vi "String to Type.vi"(7 "application reference (local)":refnum<vi>, 8 "Error In":errorcluster, 11 "String":string) -> (0 "Error Out":errorcluster, 2 "Rest of the String":string, 3 "Type":variant)   [LabVIEW 2015, in "Scripting.lvlib"]
uses:
  Scripting.lvlib
  <vilib>/Utility/Data Type/Type Definitions/Data Type.ctl
  <vilib>/fxp/LVFixedPointRepBitsTypeDef.ctl
  <vilib>/fxp/LVFixedPointRepRangeTypeDef.ctl
  <vilib>/Utility/Data Type/Type Definitions/Refnum Type.ctl
  <vilib>/Utility/Data Type/Type Definitions/VI Info.ctl
  <vilib>/Utility/Data Type/Type Definitions/Tag Type.ctl
  <vilib>/Utility/Data Type/NI_Data Type.lvlib
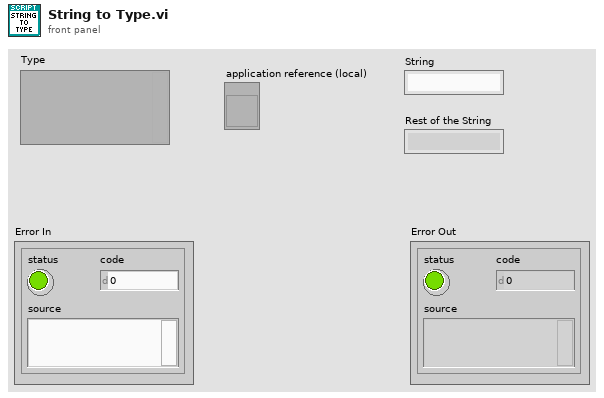
[diagram p1: front panel]
types:
  T1 = typedef "NI_Data Type.lvlib/Data Type.ctl" = enum8{"Invalid Type", "Void", "I8", "I16", "I32", "I64", "U8", "U16", "U32", "U64", "Single Float", "Double Float", "Extended Float", "Single Complex", "Double Complex", "Extended Complex", "Enum U8", "Enum U16", "Enum U32", "Enum U64", "Single Float With Unit", "Double Float With Unit", "Extended Float With Unit", "Single Complex with Unit", "Double Complex with Unit", "Extended Complex with Unit", "Boolean", "String", "Path", "Picture", "Tag", "Array", "Cluster", "Variant", "LV Variant", "Waveform", "Timestamp", "Digital Waveform", "Digital Data", "ExpressData", "Refnum", "External Data", "VI", "Poly VI", "LabVIEW Class Instance", "Fixed Point"}
  T2 = cluster{"Unit Type":enum8{"Radians", "Steradians", "Seconds", "Meters", "Kilograms", "Amperes", "Kelvins", "Moles", "Candelas", "InvalidUnit"}, "Exponent":i8}[]
  T3 = typedef "LVFixedPointRepBitsTypeDef.ctl" = cluster{"Signed":bool, "Word Length":u32, "Integer Word Length":i32}
  T4 = typedef "LVFixedPointRepRangeTypeDef.ctl" = cluster{"Range Min":dbl, "Range Max":dbl, "Delta":dbl}
  T5 = cluster{"FXP Representation":T3, "FXP Range":T4, "Include Overflow Status?":bool}
  T6 = typedef "NI_Data Type.lvlib/Refnum Type.ctl" = enum16{"NotARefnum", "UnknownRefnum", "Generic", "Datalog", "ByteStream", "Device", "Occurence", "TCPNetConnection", "Auto", "Menu", "Imaq", "Hardware", "DataSocket", "Visa", "IVI", "UDPNetConnection", "Notifier", "Queue", "Irda", "EventReg", "DotNet", "UserEvent", "Callback", "UNUSED_EMPTY_POSITION", "BlueToothNetConnection", "LVObjApp", "LVObjVI", "LVObjUnknown", "GenericClass", "UserDefinedRefnumTag", "DataValue", "RT FIFO", "TDMS File"}
  T7 = typedef "NI_Data Type.lvlib/VI Info.ctl" = cluster{"Connector Pane Pattern":i16, "Connector Pane Rotation":i16, "Flags":u32[], "Modification Date":timestamp, "Asynchronous":bool, "Non-Function":bool, "Subroutine":bool, "SubSystem":bool}
  T8 = typedef "NI_Data Type.lvlib/Tag Type.ctl" = enum16{"kNoTagType", "\tkDSCTagType", "\tkOldDAQTagType", "\tkIVITagType", "\tkVISATagType", "\tkGenClassTagType", "\tkUnusedTagType1", "\tkFPTagType", "\tkMotionTagType", "\tkDAQmxTaskTagType", "\tkDAQmxChannelTagType", "\tkDAQmxScaleTagType", "\tkDAQmxDeviceTagType", "\tkDAQmxTerminalTagType", "\tkDAQmxPhysChanTagType", "\tkDAQmxTriggerTagType", "\tkDAQmxSwitchTagType", "\tkDAQmxSignalTagType", "\tkUnusedTagType2", "\tkCANTaskTagType", "\tkCANInterfaceTagType", "\tkCANChannelTagType", "\tkNumTagTypes"}
  T9 = cluster{"Type":enum8{"Variable", "Fixed", "Bounded"}, "Size":u32}[]
  T10 = cluster{"string":string, string, "string":string}
  T11 = typedef "NI_Data Type.lvlib/Type Definition Info.ctl" = cluster{"Name":string, "Timestamp":u32}
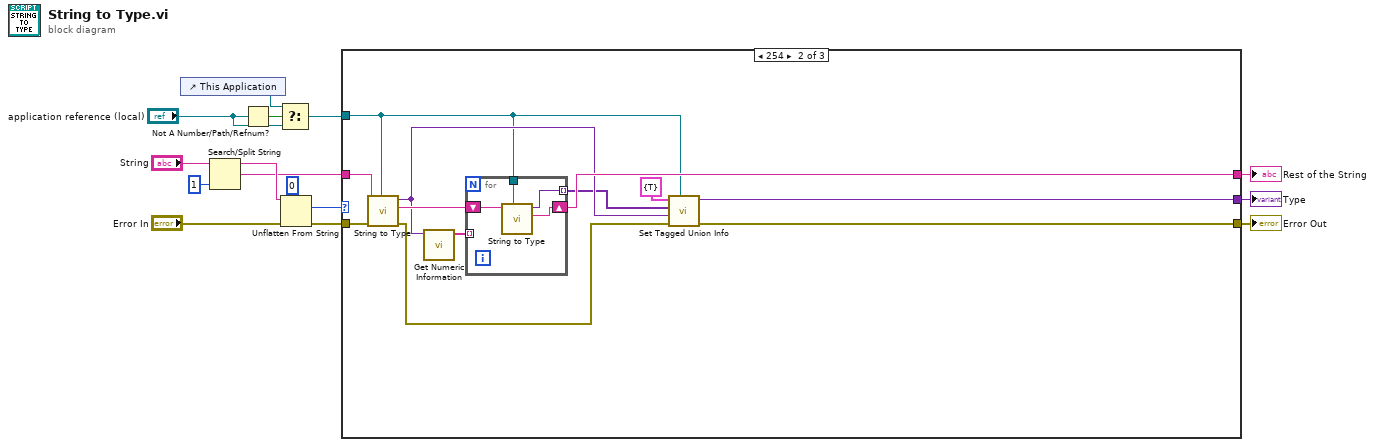
[diagram p0: block diagram]
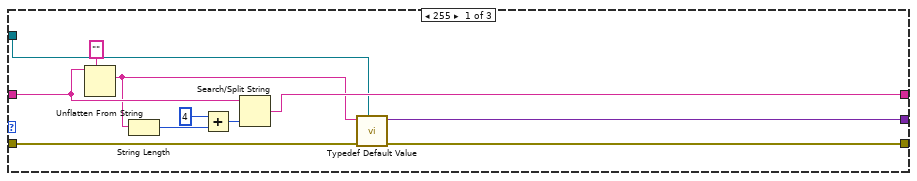
[diagram p2: hidden frame]
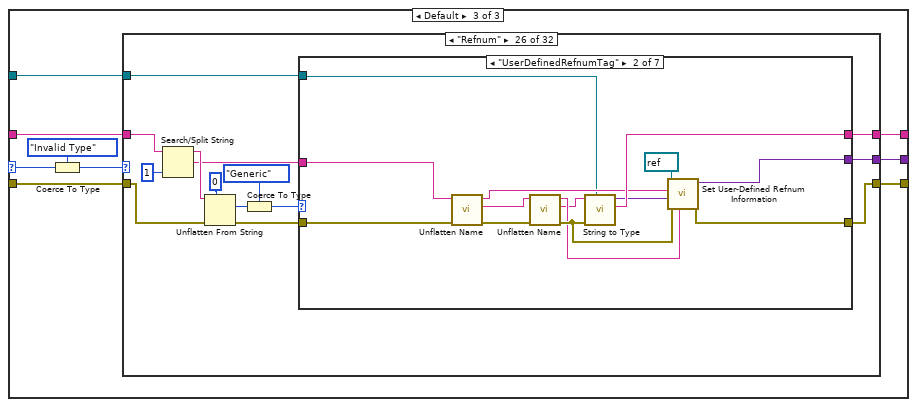
[diagram p3: hidden frame]
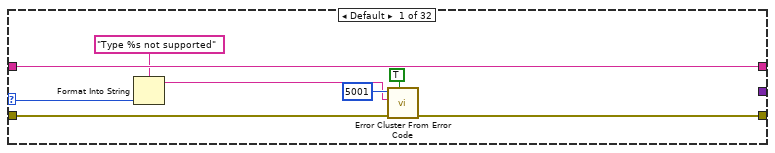
[diagram p4: hidden frame]
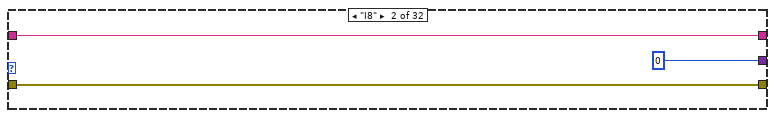
[diagram p5: hidden frame]
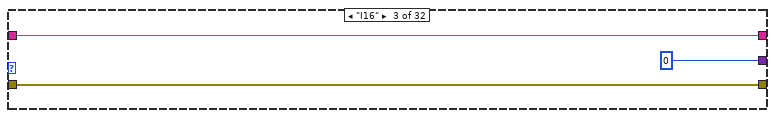
[diagram p6: hidden frame]
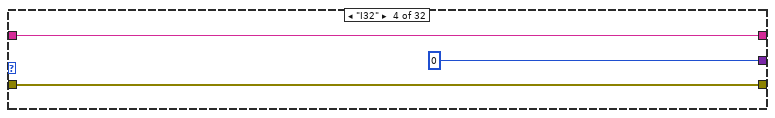
[diagram p7: hidden frame]
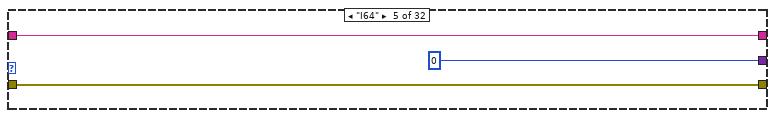
[diagram p8: hidden frame]
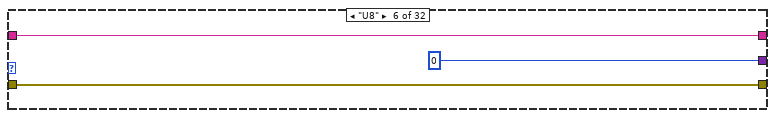
[diagram p9: hidden frame]
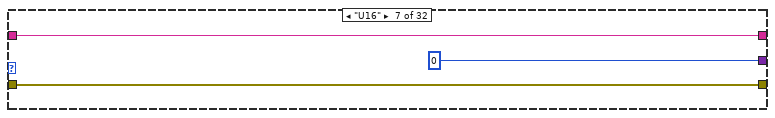
[diagram p10: hidden frame]
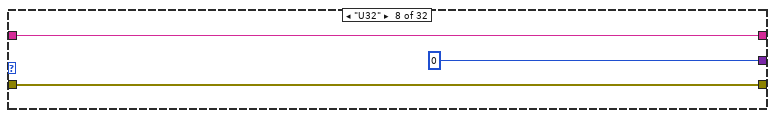
[diagram p11: hidden frame]
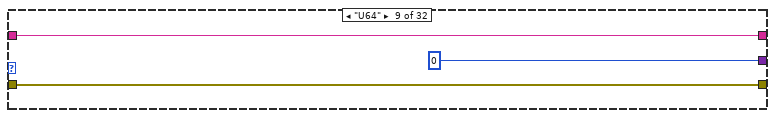
[diagram p12: hidden frame]
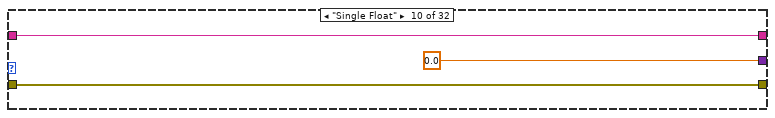
[diagram p13: hidden frame]
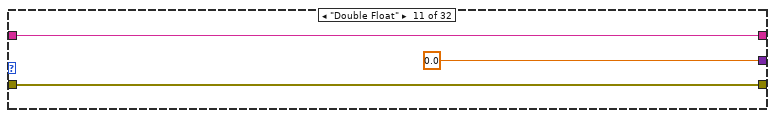
[diagram p14: hidden frame]
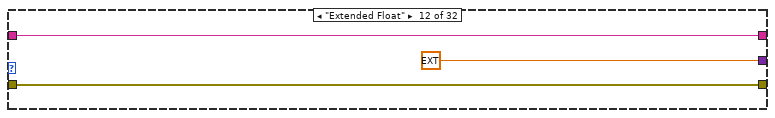
[diagram p15: hidden frame]
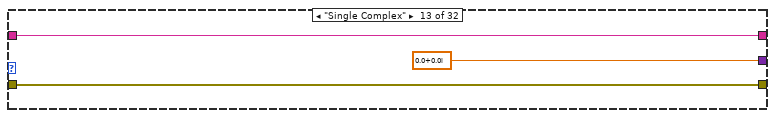
[diagram p16: hidden frame]
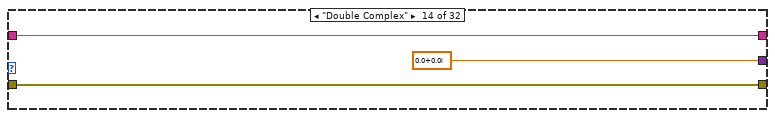
[diagram p17: hidden frame]
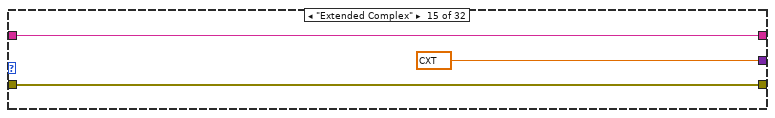
[diagram p18: hidden frame]
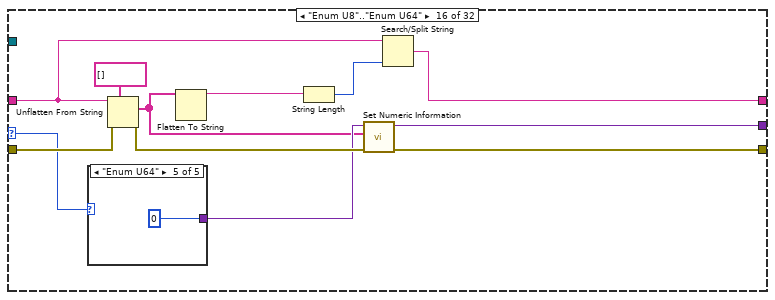
[diagram p19: hidden frame]
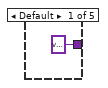
[diagram p20: hidden frame]
diagram:
  n1 = control-ref of="This Application"() -> (w3:refnum<vi>)
  n2 = Search/Split String(string="String", offset (0)=1) -> (substring before match=w8:string, match + rest of string=w6:string)  [unwired: 1 in, 1 out]
  n3 = Not A Number/Path/Refnum?(number/path/refnum="application reference (local)") -> (NaN/Path/Refnum?=w4:bool)
  n4 = Select(t=w3, s=w4, f="application reference (local)") -> (s? t:f=w2:refnum<vi>)
  n5 = Unflatten From String(type=u8 0, binary string=w8, error in (no error)="Error In") -> (value=w14:u8, error out=w12:errorcluster)  [unwired: 2 in, 1 out]
  n6 = case shown="254" w14 {
    selector: w14 -> [_ _ w51]
    tunnel: w6 -> [w20 w38 w45]
    tunnel: w12 -> [w24 w37 w48]
    tunnel: [w26 w34 w46] -> w11
    tunnel: [w25 w33 w47] -> w10
    tunnel: [w23 w32 w44] -> w5
    tunnel: w2 -> [w16 w27 w43]
    frame 255 {
      n7 = Unflatten From String(type="", binary string=w20) -> (value=w17:string)  [unwired: 3 in, 2 out]
      n8 = String Length(string=w17) -> (length=w21:i32)
      n9 = Add(x=4, y=w21) -> (x+y=w19:i32)
      n10 = Search/Split String(string=w20, offset (0)=w19) -> (match + rest of string=w23:string)  [unwired: 1 in, 2 out]
      n11 = call "Typedef Default Value.vi"("application reference (local)"=w16, "error in (no error)"=w24, "Name"=w17) -> ("error out"=w25:errorcluster, "Value"=w26:variant)  [unwired: 7 in]
    }
    frame 254 {
      n12 = call "String to Type.vi"("application reference (local)"=w27, "Error In"=w37, "String"=w38) -> ("Error Out"=w30:errorcluster, "Rest of the String"=w35:string, "Type"=w31:variant)  [unwired: 6 in]
      n13 = call <vilib>:"Get Numeric Information.vi"("Variant"=w31) -> ("Enum Names"=w36:string[])  [unwired: 7 in, 3 out]
      n14 = for {
        tunnel: w36 -> [_] mode=indexing
        shift-right: [w41] -> w32
        shift-left: w35 -> [w42]
        tunnel: [w40] -> w29 mode=indexing
        tunnel: w27 -> [w39]
        n15 = call "String to Type.vi"("application reference (local)"=w39, "String"=w42) -> ("Rest of the String"=w41:string, "Type"=w40:variant)  [unwired: 7 in, 1 out]
      }
      n16 = call "Set Tagged Union Info.vi"("application reference (local)"=w27, "error in (no error)"=w30, "Enum Type"=w31, "Element Types"=w29, "Variant in"=cluster{bool} {TRUE}) -> ("error out"=w33:errorcluster, "Variant out"=w34:variant)  [unwired: 5 in]
    }
    frame Default {
      n17 = Coerce To Type(0:w51, 1:Data_Type."Invalid Type" ("Type")) -> (2:w49:T1)
      n18 = case shown="\"Refnum\"" w49 {
        selector: w49 -> [w54 _ _ _ _ _ _ _ _ _ _ _ _ _ _ w108 w128 _ _ _ _ _ _ _ _ _ _ _ _ _ _ _]
        tunnel: w48 -> [w55 w62 w65 w68 w71 w74 w77 w80 w83 w86 w89 w92 w95 w98 w101 w112 w132 w153 w156 w159 w162 w165 w168 w171 w174 w186 w287 w305 w323 w339 w363 w379]
        tunnel: [w58 w62 w65 w68 w71 w74 w77 w80 w83 w86 w89 w92 w95 w98 w101 w110 w130 w147 w156 w159 w162 w165 w168 w171 w174 w183 w284 w305 w316 w341 w348 w369] -> w47
        tunnel: [_ i8 0 i16 0 0 i64 0 u8 0 u16 0 u32 0 u64 0 sgl 0.0 0.0 ext 0.0 csg 0.0+0.0i cdb 0.0+0.0i cxt 0.0+0.0i w109 w129 w148 FALSE "" path "" picture data[5B] ("new picture") timestamp(0 s since 1904-01-01) ("Time Stamp") digitalwaveform {"t0"=timestamp(0 s since 1904-01-01), "dt"=0.0, "Y"={"transitions"=[], "data"=[]}} ("output waveform") digitaldata {"transitions"=[], "data"=[]} ("output waveform") w180 w281 w302 w317 w340 w346 w368] -> w46
        tunnel: w45 -> [w59 w60 w63 w66 w69 w72 w75 w78 w81 w84 w87 w90 w93 w96 w99 w104 w125 w140 w154 w158 w161 w164 w167 w170 w173 w181 w282 w304 w321 w335 w364 w378]
        tunnel: [w59 w60 w63 w66 w69 w72 w75 w78 w81 w84 w87 w90 w93 w96 w99 w102 w123 w150 w154 w158 w161 w164 w167 w170 w173 w182 w283 w304 w307 w344 w365 w372] -> w44
        tunnel: w43 -> [_ _ _ _ _ _ _ _ _ _ _ _ _ _ _ _ _ _ _ _ _ _ _ _ _ w175 _ _ w306 _ w345 w366]
        frame Default {
          n19 = Format Into String(format string="Type %s not supported", w54) -> (resulting string=w52:string)  [unwired: 2 in, 1 out]
          n20 = call <vilib>:"Error Cluster From Error Code.vi"("show call chain? (False)"=TRUE, "error in (no error)"=w55, "error message (\"\")"=w52, "error code (0)"=5001) -> ("error out"=w58:errorcluster)  [unwired: 5 in]
        }
        frame "I8" {
        }
        frame "I16" {
        }
        frame "I32" {
        }
        frame "I64" {
        }
        frame "U8" {
        }
        frame "U16" {
        }
        frame "U32" {
        }
        frame "U64" {
        }
        frame "Single Float" {
        }
        frame "Double Float" {
        }
        frame "Extended Float" {
        }
        frame "Single Complex" {
        }
        frame "Double Complex" {
        }
        frame "Extended Complex" {
        }
        frame "Enum U8".."Enum U64" {
          n21 = case shown="\"Enum U64\"" w108 {
            tunnel: [variant u8 0 u16 0 u32 0 u64 0] -> w107
            frame Default {
            }
            frame "Enum U8" {
            }
            frame "Enum U16" {
            }
            frame "Enum U32" {
            }
            frame "Enum U64" {
            }
          }
          n22 = Unflatten From String(type=string[] [], binary string=w104, error in (no error)=w112) -> (value=w106:string[], error out=w111:errorcluster)  [unwired: 2 in, 1 out]
          n23 = Flatten To String(anything=w106) -> (data string=w105:string)  [unwired: 3 in, 2 out]
          n24 = String Length(string=w105) -> (length=w103:i32)
          n25 = call <vilib>:"Set Numeric Information.vi"("error in (no error)"=w111, "Enum Names"=w106, "Variant in"=w107) -> ("error out"=w110:errorcluster, "Variant out"=w109:variant)  [unwired: 7 in]
          n26 = Search/Split String(string=w104, offset (0)=w103) -> (match + rest of string=w102:string)  [unwired: 1 in, 2 out]
        }
        frame "Single Float With Unit".."Extended Complex with Unit" {
          n27 = Concatenate Strings("\u0000\u0000\u0000" ("string"), w125) -> (w120:string)
          n28 = Unflatten From String(type=T2 [], binary string=w120, error in (no error)=w132) -> (value=w121:T2, error out=w131:errorcluster)  [unwired: 2 in, 1 out]
          n29 = case shown="\"Extended Complex with Unit\"" w128 {
            tunnel: [variant sgl 0.0 0.0 ext 0.0 csg 0.0+0.0i cdb 0.0+0.0i cxt 0.0+0.0i] -> w127
            frame Default {
            }
            frame "Single Float With Unit" {
            }
            frame "Double Float With Unit" {
            }
            frame "Extended Float With Unit" {
            }
            frame "Single Complex with Unit" {
            }
            frame "Double Complex with Unit" {
            }
            frame "Extended Complex with Unit" {
            }
          }
          n30 = Flatten To String(anything=w121) -> (data string=w126:string)  [unwired: 3 in, 2 out]
          n31 = String Length(string=w126) -> (length=w124:i32)
          n32 = call <vilib>:"Set Numeric Information.vi"("error in (no error)"=w131, "Units"=w121, "Variant in"=w127) -> ("error out"=w130:errorcluster, "Variant out"=w129:variant)  [unwired: 7 in]
          n33 = Search/Split String(string=w120, offset (0)=w124) -> (match + rest of string=w123:string)  [unwired: 1 in, 2 out]
        }
        frame "Fixed Point" {
          n34 = Unflatten From String(type=T5 {"FXP Representation"={"Signed"=FALSE, "Word Length"=0, "Integer Word Length"=0}, "FXP Range"={"Range Min"=0.0, "Range Max"=0.0, "Delta"=0.0}, "Include Overflow Status?"=FALSE} ("output cluster"), binary string=w140, error in (no error)=w153) -> (value=w145:T5, error out=w146:errorcluster)  [unwired: 2 in, 1 out]
          n35 = Unbundle(w145) -> ("FXP Representation"=w144:T3, "FXP Range"=w143:T4, "Include Overflow Status?"=w142:bool)
          n36 = Flatten To String(anything=w145) -> (data string=w152:string)  [unwired: 3 in, 2 out]
          n37 = String Length(string=w152) -> (length=w151:i32)
          n38 = Search/Split String(string=w140, offset (0)=w151) -> (match + rest of string=w150:string)  [unwired: 1 in, 2 out]
          n39 = call <vilib>:"Set Fixed-Point Information.vi"("Include Overflow Status?"=w142, "error in (no error)"=w146, "FXP Range"=w143, "FXP Representation"=w144, "Variant in"=fxp<+,1,1> 0.0) -> ("error out"=w147:errorcluster, "Variant out"=w148:variant)  [unwired: 5 in]
        }
        frame "Boolean" {
        }
        frame "String" {
        }
        frame "Path" {
        }
        frame "Picture" {
        }
        frame "Timestamp" {
        }
        frame "Digital Waveform" {
        }
        frame "Digital Data" {
        }
        frame "Refnum" {
          n40 = Search/Split String(string=w181, offset (0)=1) -> (substring before match=w188:string, match + rest of string=w185:string)  [unwired: 1 in, 1 out]
          n41 = Unflatten From String(type=u8 0, binary string=w188, error in (no error)=w186) -> (value=w179:u8, error out=w184:errorcluster)  [unwired: 2 in, 1 out]
          n42 = Coerce To Type(0:w179, 1:Refnum_Type."Generic" ("Reference Type")) -> (2:w178:T6)
          n43 = case shown="\"UserDefinedRefnumTag\"" w178 {
            selector: w178 -> [w192 _ _ w242 _ _ w270]
            tunnel: w185 -> [w195 w210 w222 w246 w256 w259 w272]
            tunnel: w184 -> [w197 w211 w227 w245 w255 w258 w275]
            tunnel: [w198 w212 w217 w241 w255 w258 w276] -> w183
            tunnel: [w194 w208 w223 w246 w256 w259 w274] -> w182
            tunnel: [w190 w201 w214 w247 refnum<k31> refnum ("connection ID out") refnum<visa-resource-name> refnum ("VISA resource name out") w273] -> w180
            tunnel: w175 -> [w189 w199 w213 _ _ _ w260]
            frame "Datalog", "Notifier", "Queue", "DataValue" {
              n44 = call "String to Type.vi"("application reference (local)"=w189, "Error In"=w197, "String"=w195) -> ("Error Out"=w196:errorcluster, "Rest of the String"=w194:string, "Type"=w193:variant)  [unwired: 6 in]
              n45 = call <vilib>:"Set Refnum Information.vi"("error in (no error)"=w196, "Strict Type"=w193, "Reference Type"=w192, "Variant in"=refnum<data-value> refnum ("data value reference")) -> ("error out"=w198:errorcluster, "Variant out"=w190:variant)  [unwired: 6 in]
            }
            frame "UserDefinedRefnumTag" {
              n46 = call "Unflatten Name.vi"("error in (no error)"=w211, "Data String"=w210) -> ("error out"=w209:errorcluster, "Rest of String"=w203:string, "Name"=w204:string)  [unwired: 7 in]
              n47 = call "Unflatten Name.vi"("error in (no error)"=w209, "Data String"=w203) -> ("error out"=w207:errorcluster, "Rest of String"=w202:string, "Name"=w205:string)  [unwired: 7 in]
              n48 = call "String to Type.vi"("application reference (local)"=w199, "Error In"=w207, "String"=w202) -> ("Rest of the String"=w208:string, "Type"=w206:variant)  [unwired: 6 in, 1 out]
              n49 = call <vilib>:"Set User-Defined Refnum Information.vi"("Type Name"=w205, "error in (no error)"=w207, "User Data"=w206, "Class Name"=w204, "Variant in"=refnum<k21> refnum ("task out")) -> ("error out"=w212:errorcluster, "Variant out"=w201:variant)  [unwired: 5 in]
            }
            frame "LVObjVI" {
              w216 = refnum<vi> refnum
              n50 = Unflatten From String(type=T7 {"Connector Pane Pattern"=0, "Connector Pane Rotation"=0, "Flags"=[], "Modification Date"=timestamp(0 s since 1904-01-01), "Asynchronous"=FALSE, "Non-Function"=FALSE, "Subroutine"=FALSE, "SubSystem"=FALSE} ("VI Info"), binary string=w222, error in (no error)=w227) -> (value=w235:T7, error out=w234:errorcluster)  [unwired: 2 in, 1 out]
              n51 = Flatten To String(anything=w235) -> (data string=w229:string)  [unwired: 3 in, 2 out]
              n52 = String Length(string=w229) -> (length=w230:i32)
              n53 = Search/Split String(string=w222, offset (0)=w230) -> (match + rest of string=w231:string)  [unwired: 1 in, 2 out]
              n54 = Search/Split String(string=w231, offset (0)=1) -> (substring before match=w226:string, match + rest of string=w221:string)  [unwired: 1 in, 1 out]
              n55 = Unflatten From String(type=u8 0, binary string=w226, error in (no error)=w234) -> (value=w224:u8, error out=w220:errorcluster)  [unwired: 2 in, 1 out]
              n56 = for {
                N: w224 -> [_]
                tunnel: [w239] -> w225 mode=indexing
                shift-right: [w238] -> w223
                shift-left: w221 -> [w240]
                tunnel: [w237] -> _ mode=indexing
                tunnel: w213 -> [w236]
                n57 = call "String to Type.vi"("application reference (local)"=w236, "String"=w240) -> ("Error Out"=w237:errorcluster, "Rest of the String"=w238:string, "Type"=w239:variant)  [unwired: 7 in]
              }
              n58 = call <vilib>:"Set VI Information.vi"("error in (no error)"=w220, "VI Terminal Types"=w225, "VI Info"=w235, "Variant in"=w216) -> ("error out"=w218:errorcluster, "Variant out"=w219:variant)  [unwired: 6 in]
              n59 = call <vilib>:"Set Refnum Information.vi"("error in (no error)"=w218, "Strict Type"=w219, "Reference Type"=Refnum_Type."LVObjVI", "Variant in"=w216) -> ("error out"=w217:errorcluster, "Variant out"=w214:variant)  [unwired: 6 in]
            }
            frame Default {
              n60 = call <vilib>:"Set Refnum Information.vi"("error in (no error)"=w245, "Reference Type"=w242, "Variant in"=refnum<k4> refnum ("occurrence")) -> ("error out"=w243:errorcluster, "Variant out"=w247:variant)  [unwired: 7 in]
              n61 = case shown="Error" w243 {
                tunnel: w242 -> [_ w249]
                tunnel: [_ w248] -> w241
                frame No Error {
                }
                frame Error {
                  n62 = Format Into String(format string="Type %s not supported", w249) -> (resulting string=w250:string)  [unwired: 2 in, 1 out]
                  n63 = call <vilib>:"Error Cluster From Error Code.vi"("show call chain? (False)"=TRUE, "error message (\"\")"=w250, "error code (0)"=5001) -> ("error out"=w248:errorcluster)  [unwired: 6 in]
                }
              }
            }
            frame "BlueToothNetConnection" {
            }
            frame "Visa" {
            }
            frame "UserEvent" {
              n64 = call "Unflatten Name.vi"("error in (no error)"=w275, "Data String"=w272) -> ("error out"=w271:errorcluster, "Rest of String"=w264:string, "Name"=w269:string)  [unwired: 7 in]
              n65 = call "String to Type.vi"("application reference (local)"=w260, "Error In"=w271, "String"=w269) -> ("Error Out"=w265:errorcluster, "Rest of the String"=w274:string, "Type"=w266:variant)  [unwired: 6 in]
              n66 = call <vilib>:"Get Type Information.vi"("error in (no error)"=w265, "Variant"=w266) -> ("error out"=w268:errorcluster, "Type Definition Info"=w267:T11)  [unwired: 5 in, 3 out]
              n67 = call <vilib>:"Set Type Information.vi"("error in (no error)"=w268, "Type Definition Info"=w267, "Name"=w264, "Variant in"=w266) -> ("error out"=w262:errorcluster, "Variant out"=w263:variant)  [unwired: 6 in]
              n68 = call <vilib>:"Set Refnum Information.vi"("error in (no error)"=w262, "Strict Type"=w263, "Reference Type"=w270, "Variant in"=refnum<user-event> refnum) -> ("error out"=w276:errorcluster, "Variant out"=w273:variant)  [unwired: 6 in]
            }
          }
        }
        frame "Tag" {
          n69 = Search/Split String(string=w282, offset (0)=1) -> (substring before match=w289:string, match + rest of string=w286:string)  [unwired: 1 in, 1 out]
          n70 = Unflatten From String(type=u8 0, binary string=w289, error in (no error)=w287) -> (value=w280:u8, error out=w285:errorcluster)  [unwired: 2 in, 1 out]
          n71 = Coerce To Type(0:w280, 1:Tag_Type."kNoTagType" ("Tag Type")) -> (2:w277:T8)
          n72 = case shown="Default" w277 {
            selector: w277 -> [w293 _]
            tunnel: w286 -> [w298 w301]
            tunnel: w285 -> [w292 w299]
            tunnel: [w291 w299] -> w284
            tunnel: [w298 w301] -> w283
            tunnel: [variant ("Variant out") tag "" ("physical channels")] -> w281
            frame Default {
              n73 = Format Into String(format string="Type %s not supported", w293) -> (resulting string=w294:string)  [unwired: 2 in, 1 out]
              n74 = call <vilib>:"Error Cluster From Error Code.vi"("show call chain? (False)"=TRUE, "error in (no error)"=w292, "error message (\"\")"=w294, "error code (0)"=5001) -> ("error out"=w291:errorcluster)  [unwired: 5 in]
            }
            frame "\tkDAQmxPhysChanTagType" {
            }
          }
        }
        frame "Variant", "LV Variant" {
          n75 = To Variant(anything=variant ("Variant out")) -> (Variant=w302:variant)
        }
        frame "Array" {
          n76 = Concatenate Strings("\u0000\u0000\u0000" ("string"), w321) -> (w311:string)
          n77 = Unflatten From String(type=T9 [] ("Array Lengths"), binary string=w311, error in (no error)=w323) -> (value=w309:T9, error out=w319:errorcluster)  [unwired: 2 in, 1 out]
          n78 = Flatten To String(anything=w309, error in (no error)=w319) -> (data string=w322:string, error out=w314:errorcluster)  [unwired: 2 in, 1 out]
          n79 = String Length(string=w322) -> (length=w320:i32)
          n80 = Search/Split String(string=w311, offset (0)=w320) -> (match + rest of string=w308:string)  [unwired: 1 in, 2 out]
          n81 = call "String to Type.vi"("application reference (local)"=w306, "Error In"=w314, "String"=w308) -> ("Error Out"=w313:errorcluster, "Rest of the String"=w307:string, "Type"=w315:variant)  [unwired: 6 in]
          n82 = call <vilib>:"Set Array Information.vi"("error in (no error)"=w313, "Array Lengths"=w309, "Array Element"=w315, "Variant in"=bool[] []) -> ("error out"=w316:errorcluster, "Variant out"=w317:variant)  [unwired: 6 in]
        }
        frame "LabVIEW Class Instance" {
          n83 = Unflatten From String(type=T10 {"string"="", "", "string"=""} ("output cluster"), binary string=w335) -> (value=w333:T10)  [unwired: 3 in, 2 out]
          n84 = Flatten To String(anything=w333) -> (data string=w332:string)  [unwired: 3 in, 2 out]
          n85 = Unbundle(w333) -> ("string"=w329:string, w328:string, "string"=w327:string)
          n86 = String Length(string=w332) -> (length=w331:i32)
          n87 = Concatenate Strings(w329, w328, w327) -> (w326:string)
          n88 = Search/Split String(string=w335, offset (0)=w331) -> (match + rest of string=w344:string)  [unwired: 1 in, 2 out]
          n89 = String To Byte Array(string=w326) -> (unsigned byte array=w325:u8[])
          n90 = Decimate 1D Array(w325) -> (w343:u8[], w342:u8[])
          n91 = Join Numbers(hi=w343, lo=w342) -> ((hi.lo)=w334:u16[])
          n92 = To Word Integer(number=w334) -> (16bit integer=w324:i16[])
          n93 = call <vilib>:"Get LV Class Default Value By Name.vi"("error in (no error)"=w339, "class name"=w328) -> ("error out"=w336:errorcluster, "object"=w338:refnum<class>)  [unwired: 8 in]
          n94 = Variant To Flattened String(Variant=w338) -> (data string=w337:string)  [unwired: 1 out]
          n95 = Flattened String To Variant(4:w336, 6:w337, 7:w324) -> (0:w341:errorcluster, 3:w340:variant)
        }
        frame "Waveform" {
          w358 = 31 ("index")
          n96 = call "String to Type.vi"("application reference (local)"=w345, "Error In"=w363, "String"=w364) -> ("Error Out"=w349:errorcluster, "Rest of the String"=w365:string, "Type"=w347:variant)  [unwired: 6 in]
          n97 = Variant To Flattened String(Variant=waveform(dbl) {"t0"=timestamp(0 s since 1904-01-01), "dt"=1.0, "Y"=[]} ("Waveform")) -> (data string=w350:string, 1:w361:i16[])
          n98 = Delete From Array(array=w361, length=2, index=w358) -> (array with subset deleted=w359:i16[])  [unwired: 1 out]
          n99 = Variant To Flattened String(Variant=w347) -> (1:w357:i16[])  [unwired: 1 out]
          n100 = Insert Into Array(array=w359, index=w358, new element=w357) -> (w353:i16[])
          n101 = Array Size(array=w353) -> (size(s)=w356:i32)
          n102 = Multiply(x=w356, y=2) -> (x*y=w354:i32)
          n103 = Replace Array Subset(array=w353, new element=w354, index=0) -> (w351:i16[])
          n104 = Flattened String To Variant(4:w349, 6:w350, 7:w351) -> (0:w348:errorcluster, 3:w346:variant)
        }
        frame "Cluster" {
          n105 = Search/Split String(string=w378, offset (0)=2) -> (match + rest of string=w374:string)  [unwired: 1 in, 2 out]
          n106 = Unflatten From String(type=i16 0, binary string=w378, error in (no error)=w379) -> (value=w375:i16, error out=w373:errorcluster)  [unwired: 2 in, 1 out]
          n107 = for {
            N: w375 -> [_]
            shift-right: [w381] -> w371
            shift-left: w373 -> [w394]
            shift-right: [w386] -> w372
            shift-left: w374 -> [w393]
            tunnel: [w384] -> w370 mode=indexing
            tunnel: w366 -> [w380]
            n108 = Unflatten From String(type=i8 0, binary string=w393, error in (no error)=w394) -> (value=w389:i8, error out=w387:errorcluster)  [unwired: 2 in, 1 out]
            n109 = Search/Split String(string=w393, offset (0)=1) -> (match + rest of string=w390:string)  [unwired: 1 in, 2 out]
            n110 = Search/Split String(string=w390, offset (0)=w389) -> (substring before match=w383:string, match + rest of string=w388:string)  [unwired: 1 in, 1 out]
            n111 = call "String to Type.vi"("application reference (local)"=w380, "Error In"=w387, "String"=w388) -> ("Error Out"=w382:errorcluster, "Rest of the String"=w386:string, "Type"=w385:variant)  [unwired: 6 in]
            n112 = call "Set Name.vi"("error in (no error)"=w382, "Name"=w383, "Type in"=w385) -> ("error out"=w381:errorcluster, "Type out"=w384:variant)  [unwired: 7 in]
          }
          n113 = call <vilib>:"Set Cluster Information.vi"("error in (no error)"=w371, "Cluster Elements"=w370, "Variant in"=cluster{bool} {FALSE}) -> ("error out"=w369:errorcluster, "Variant out"=w368:variant)  [unwired: 7 in]
        }
      }
    }
  }
  "Type" <- w11
  "Error Out" <- w10
  "Rest of the String" <- w5
